vi "AgPSA _GetMarkerMeasurement.vi"(5 "Cal?":bool, 6 "Cal Route":string[](array[string])=["", "", ""], 7 "Active Marker (1: Marker1)":u16(ring)=1 items=["Marker1"=1, "Marker2"=2, "Marker3"=3, "Marker4"=4], 8 "error in (no error)":errorcluster, 10 "Cal Freq (Hz)":dbl=100000000.0 format="%.2p", 11 "PSA In":refnum<visa-resource-name>) -> (0 "error out":errorcluster, 1 "Calibrated Marker Amplitude":dbl, 2 "Marker Position":dbl, 3 "Marker Amplitude":dbl)   [LabVIEW 2015]
uses:
  <instrlib>/Agilent ESA PSA Series/Agilent ESA PSA Series.lvlib
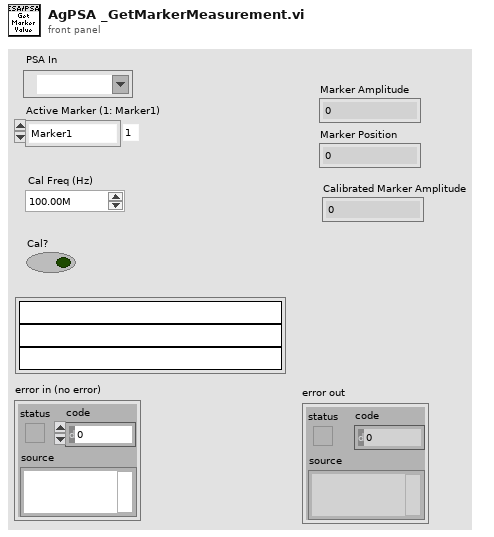
[diagram p1: front panel]
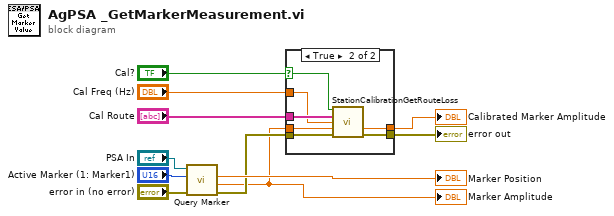
[diagram p0: block diagram]
diagram:
  n1 = call <instrlib>:"Query Marker.vi"("error in (no error)"="error in (no error)", "Active Marker (1: Marker1)"="Active Marker (1: Marker1)", "VISA resource name"="PSA In") -> ("error out"=w5:errorcluster, "Marker Amplitude"=w2:dbl, "Marker Position"=→"Marker Position":dbl)  [unwired: 5 in, 1 out]
  "Marker Amplitude" <- w2
  n2 = case shown="True" "Cal?" {
    selector: "Cal?" -> [_ w18]
    tunnel: [w12 w14] -> w1
    tunnel: [w13 w19] -> w4
    tunnel: w5 -> [w13 w20]
    tunnel: w2 -> [w12 w15]
    tunnel: "Cal Route" -> [_ w17]
    tunnel: "Cal Freq (Hz)" -> [_ w16]
    frame False {
    }
    frame True {
      n3 = call "StationCalibrationGetRouteLoss.vi"("Calibration Enabled"=w18, "Route Names"=w17, "Frequency"=w16, "Power Level"=w15, "error in (no error)"=w20) -> ("Adjusted Power Level"=w14:dbl, "error out"=w19:errorcluster)  [unwired: 7 in, 2 out]
    }
  }
  "error out" <- w4
  "Calibrated Marker Amplitude" <- w1
